vi "User Interface.vi"() -> ()   [LabVIEW 2017, in "Single Computer PvP.lvclass"]
uses:
  Single Computer PvP.lvclass
panel:
  out "Array":bool[](array[boolean])
  out "Boolean":bool
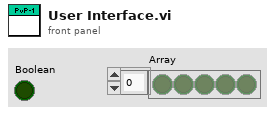
[diagram p1: front panel]
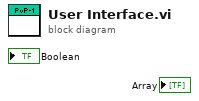
[diagram p0: block diagram]
diagram:
